vi "Varient_Current_Status.vi"(7 "Enum":enum16{"Write", "Read"}(ring), 8 "error in":errorcluster, 9 "Current Varient Status":path, 10 "Batch Size":i32, 11 "Varient count":i32) -> (0 "error out":errorcluster, 1 "Batch Size":i32, 2 "Varient Count":i32)   [LabVIEW 2017]
uses:
  <vilib>/Utility/config.llb/Write Key (I32).vi
  <vilib>/Utility/config.llb/Read Key (I32).vi
  <vilib>/Utility/config.llb/NI_LVConfig.lvlib
panel:
  # "Varient Current Status & Count"
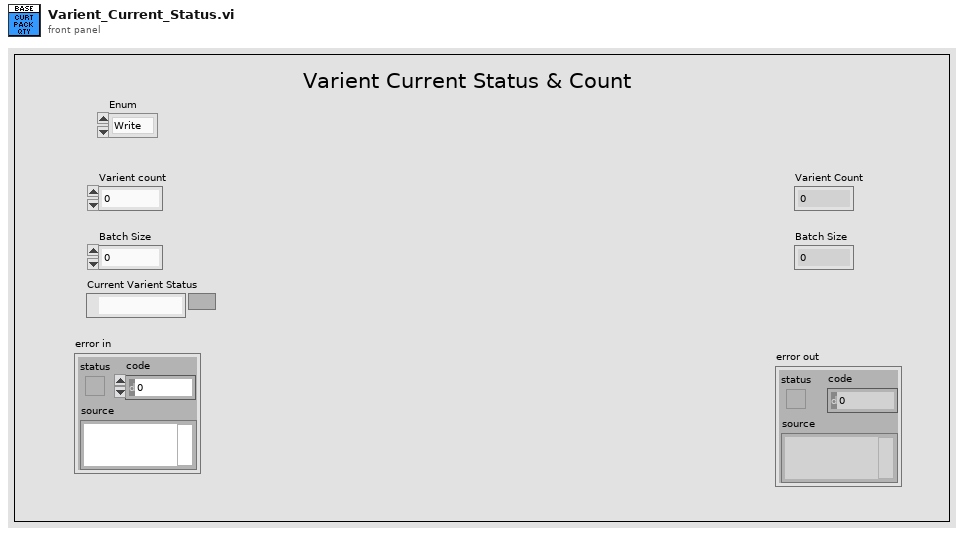
[diagram p1: front panel]
types:
  T1 = typedef "NI_LVConfig.lvlib/Config Data RefNum.ctl" = refnum<k1>
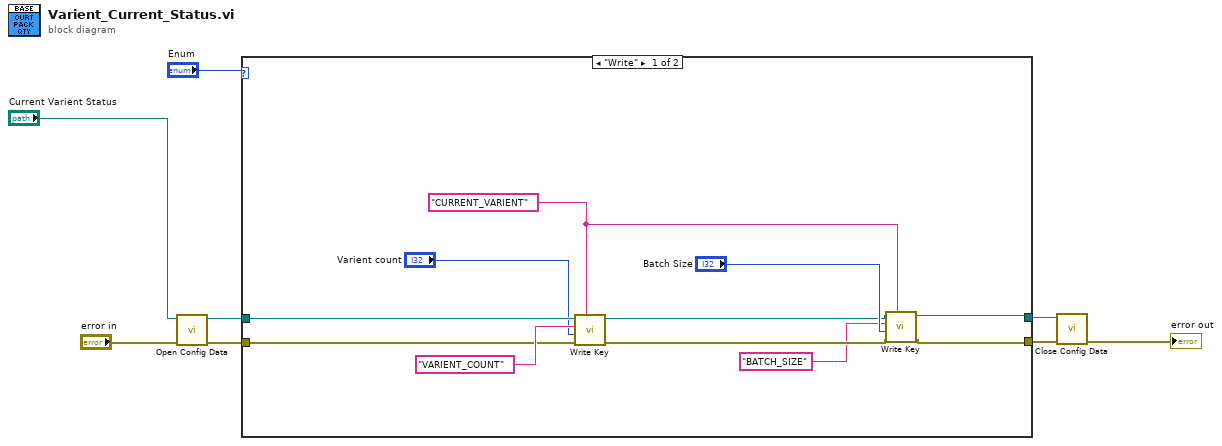
[diagram p0: block diagram]
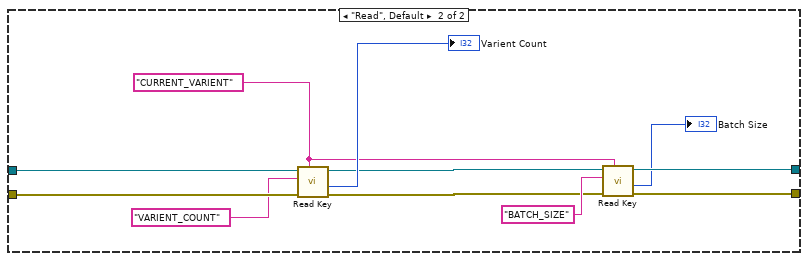
[diagram p2: hidden frame]
diagram:
  n1 = call <vilib>:"Open Config Data.vi"("error in (no error)"="error in", "configuration file path"="Current Varient Status") -> ("error out"=w7:errorcluster, "refnum"=w8:T1)  [unwired: 7 in, 1 out]
  n2 = case shown="\"Write\"" "Enum" {
    tunnel: w8 -> [w17 w30]
    tunnel: w7 -> [w18 w29]
    tunnel: [w13 w25] -> w4
    tunnel: [w11 w23] -> w3
    frame "Write" {
      w9 = "CURRENT_VARIENT" ("name or relative path")
      n3 = call-poly <vilib>:"Write Key.vi"("section"=w9, "error in (no error)"=w18, "value"="Varient count", "key"="VARIENT_COUNT" ("name or relative path"), "refnum"=w17) -> ("error out"=w14:errorcluster, "refnum out"=w12:T1)  [unwired: 4 in, 1 out]
      n4 = call-poly <vilib>:"Write Key.vi"("section"=w9, "error in (no error)"=w14, "value"="Batch Size", "key"="BATCH_SIZE" ("name or relative path"), "refnum"=w12) -> ("error out"=w13:errorcluster, "refnum out"=w11:T1)  [unwired: 4 in, 1 out]
    }
    frame "Read", Default {
      w20 = "CURRENT_VARIENT" ("name or relative path")
      n5 = call-poly <vilib>:"Read Key.vi"("section"=w20, "error in (no error)"=w29, "key"="VARIENT_COUNT" ("name or relative path"), "refnum"=w30) -> ("error out"=w26:errorcluster, "value"=→"Varient Count":i32, "refnum out"=w24:T1)  [unwired: 4 in, 1 out]
      n6 = call-poly <vilib>:"Read Key.vi"("section"=w20, "error in (no error)"=w26, "key"="BATCH_SIZE" ("name or relative path"), "refnum"=w24) -> ("error out"=w25:errorcluster, "value"=→"Batch Size":i32, "refnum out"=w23:T1)  [unwired: 4 in, 1 out]
    }
  }
  n7 = call <vilib>:"Close Config Data.vi"("error in (no error)"=w4, "refnum"=w3) -> ("error out"=→"error out":errorcluster)  [unwired: 8 in, 1 out]
